vi "Read Sync Instrument Setting.vi"(8 "error in (no error)":errorcluster, 11 "Sync Instrument configuration in":refnum<class "Synchronization configuration.lvclass">) -> (0 "error out":errorcluster, 2 "Sync Setting":T1={"Synchronization Clock"="", "DDS Clock"=0.5, "SyncDivide1"="", "SyncDivide2"="256"} {"DDS Clock" format="%#_6p"}, 3 "Sync Instrument configuration out":refnum<class "Synchronization configuration.lvclass">)   [LabVIEW 2025, in "Synchronization.lvlib" / "Synchronization configuration.lvclass"]
uses:
  Synchronization configuration.lvclass
  Sync Instrument Setting.ctl
  Synchronization configuration.lvclass/Synchronization configuration.ctl
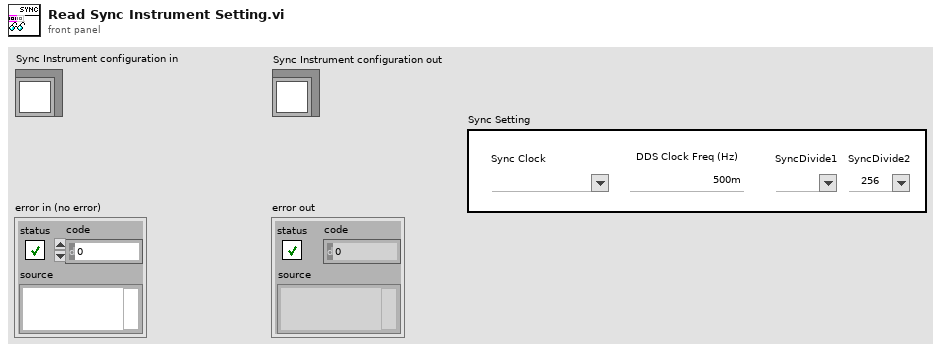
[diagram p1: front panel]
types:
  T1 = typedef "Synchronization.lvlib/Synchronization configuration.lvclass/Sync Instrument Setting.ctl" = cluster{"Synchronization Clock":string, "DDS Clock":dbl, "SyncDivide1":string, "SyncDivide2":string}
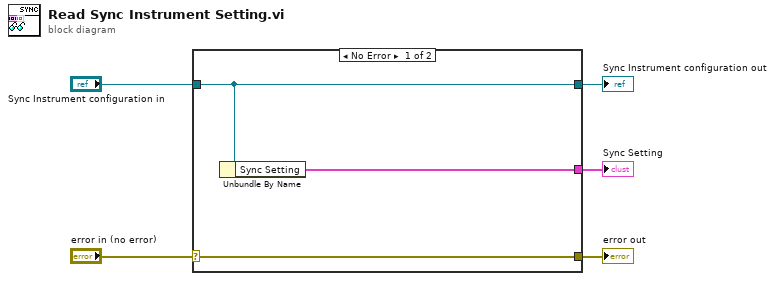
[diagram p0: block diagram]
diagram:
  n1 = case shown="No Error" "error in (no error)" {
    selector: "error in (no error)" -> [w8 w9]
    tunnel: [w8 w9] -> w4
    tunnel: [w7 w10] -> w2
    tunnel: "Sync Instrument configuration in" -> [w7 w10]
    tunnel: [w6 _] -> w1
    frame No Error {
      n2 = Unbundle By Name(w7) -> ("Sync Setting"=w6:T1)
    }
    frame Error {
    }
  }
  "error out" <- w4
  "Sync Instrument configuration out" <- w2
  "Sync Setting" <- w1
